vi "Check Disconnect.vi"(8 "error in (no error)":errorcluster, 9 "timeout in":bool, 11 "CIFTag in":refnum<class "CIF_NIChn.lvclass">) -> (0 "error out":errorcluster, 1 "timeout out":bool, 2 "Use Old Data":bool, 3 "CIFTag out":refnum<class "CIF_NIChn.lvclass">)   [LabVIEW 2021, in "CIF_NIChn.lvclass"]
uses:
  CIF_NIChn.lvclass
  D:/dev/CIF-LVCore/src/Channels/CIFChannels/CIFChannels.lvclass
  CIFChannels/Typedef/Disconnect Behavior.ctl
  CIFChannels/Typedef/Channel State.ctl
  CIFChannels/CIFChannels.lvclass/CIFChannels.ctl
  CIFChannels/Accessors/Write Channel State.vi
  CIFChannels/Accessors/Read Disconnect Behavior.vi
  CIF_NIChn.lvclass/CIF_NIChn.ctl
  CIFChannels/CIFChannels.lvclass
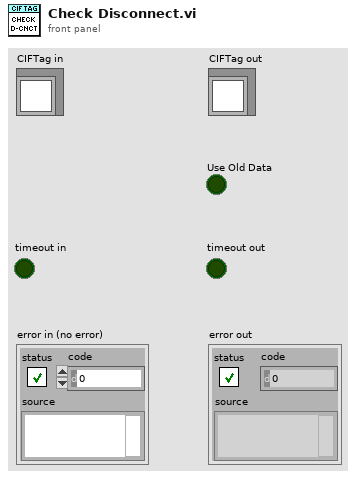
[diagram p1: front panel]
types:
  T1 = typedef "CIFChannels.lvclass/Disconnect Behavior.ctl" = enum16{"Default value", "Last value", "Error with default"}
  T2 = typedef "CIFChannels.lvclass/Channel State.ctl" = enum16{"Creating", "Disconnected", "Connecting", "Connected", "Destroyed"}
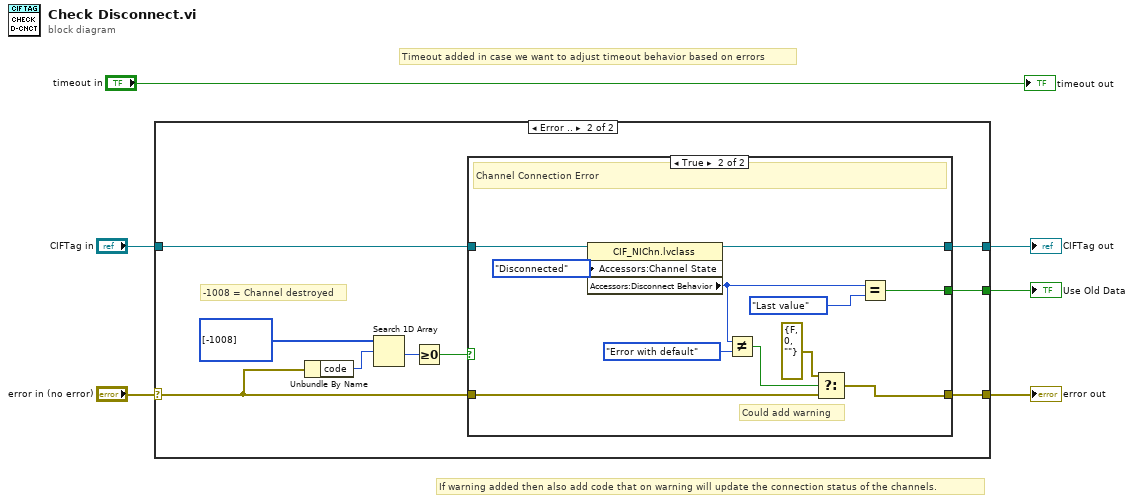
[diagram p0: block diagram]
diagram:
  # "If warning added then also add code that on warning will update the connection status of the channels."
  # "Timeout added in case we want to adjust timeout behavior based on errors"
  n1 = case shown="Error .." "error in (no error)" {
    selector: "error in (no error)" -> [w7 w9]
    tunnel: [w7 w17] -> w6
    tunnel: [w8 w16] -> w5
    tunnel: [_ w15] -> w4
    tunnel: "CIFTag in" -> [w8 w10]
    frame No Error {
    }
    frame Error {
      # "-1008 = Channel destroyed"
      n2 = Unbundle By Name(w9) -> ("code"=w11:i32)
      n3 = Search 1D Array(1D array=i32[] [-1008], element=w11) -> (index of element=w13:i32)  [unwired: 1 in]
      n4 = Greater Or Equal To 0?(x=w13) -> (x >= 0?=w12:bool)
      n5 = case shown="True" w12 {
        tunnel: w9 -> [w19 w29]
        tunnel: [w18 w23] -> w16
        tunnel: [w19 w27] -> w17
        tunnel: [_ w30] -> w15
        tunnel: w10 -> [w18 w24]
        frame False {
          # "Other error"
        }
        frame True {
          # "Could add warning"
          # "Channel Connection Error"
          n6 = property class="CIF_NIChn.lvclass"(reference=w24, "Accessors:Channel State"=Channel_State."Disconnected" ("Channel State")) -> (reference out=w23:refnum<class "CIF_NIChn.lvclass">, "Accessors:Disconnect Behavior"=w22:T1)  [unwired: 1 in, 1 out]
          n7 = Not Equal?(x=w22, y=Disconnect_Behavior."Error with default") -> (x != y?=w26:bool)
          n8 = Select(t=errorcluster {"status"=FALSE, "code"=0, "source"=""} ("f"), s=w26, f=w29) -> (s? t:f=w27:errorcluster)
          n9 = Equal?(x=w22, y=Disconnect_Behavior."Last value") -> (x = y?=w30:bool)
        }
      }
    }
  }
  "error out" <- w6
  "CIFTag out" <- w5
  "Use Old Data" <- w4
  "timeout out" <- "timeout in"
